vi "Read.vi"(8 "error in (no error)":errorcluster caption="错误输入（无错误）", 11 "6510 输入":refnum<class "6510.lvclass">) -> (0 "error out":errorcluster caption="错误输出", 2 "Measurements":dbl[](array[numeric]), 3 "6510 输出":refnum<class "6510.lvclass">)   [LabVIEW 2021, in "6510.lvclass"]
uses:
  6510.lvclass
  6510.lvclass/6510.ctl
  <instrlib>/Keithley DMM6500 DAQ6500 Series/Public/Data/Read (Multiple Points).vi
  <instrlib>/Keithley DMM6500 DAQ6500 Series/Keithley DMM6500 DAQ6500 Series.lvlib
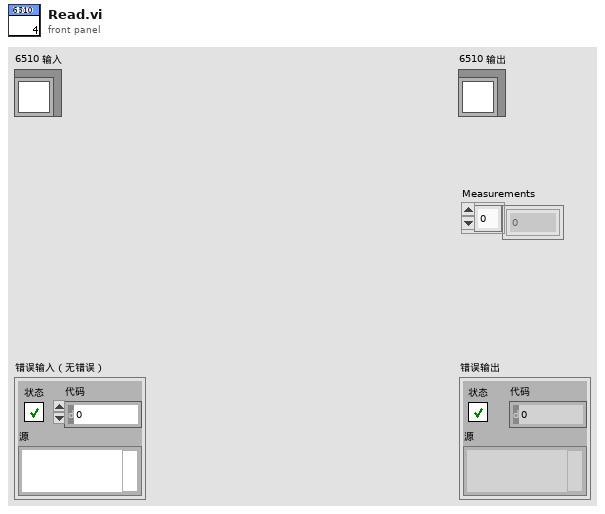
[diagram p1: front panel]
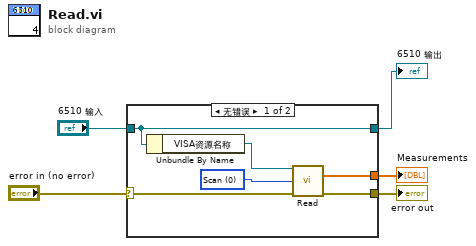
[diagram p0: block diagram]
diagram:
  n1 = case shown="无错误" "error in (no error)" {
    selector: "error in (no error)" -> [w9 w12]
    tunnel: "6510 输入" -> [w6 w13]
    tunnel: [w8 w12] -> w3
    tunnel: [w7 _] -> w2
    tunnel: [w6 w13] -> w1
    frame No Error {
      w10 = 0 items=["Scan", "Trigger"] ("Capture Mode(0: Scan)")
      n2 = Unbundle By Name(w6) -> ("VISA资源名称"=w11:refnum<visa-resource-name>)
      n3 = call-poly <instrlib>:"Read.vi"("VISA resource name"=w11, "Capture Mode(0: Scan)"=w10, "error in (no error)"=w9) -> ("Measurements"=w7:dbl[], "error out"=w8:errorcluster)  [unwired: 10 in, 1 out]
    }
    frame Error {
    }
  }
  "error out" <- w3
  "6510 输出" <- w1
  "Measurements" <- w2
